vi "Panther Logs for DQMH.vi"() -> ()   [LabVIEW 2016]
uses:
  <resource>/dialog/lvconfig.llb/LV Config Read Boolean.vi
  <resource>/dialog/lvconfig.llb/LV Config Write Boolean.vi
panel:
  in  "Panther Logs":bool
  # "Panther Logs for DQMH®\n\nThis tool creates a file called <PantherLAB_Log.csv> next to the Active LabVIEW Project.\n\nIt will create a log for each executed DQMH task .\n\n\nTo enable/disable logging click the Checkbox."
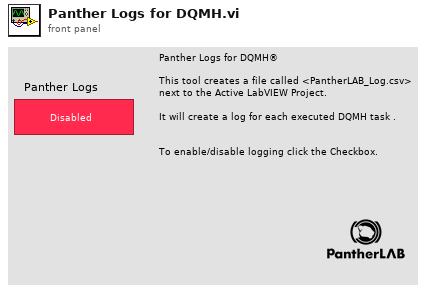
[diagram p1: front panel]
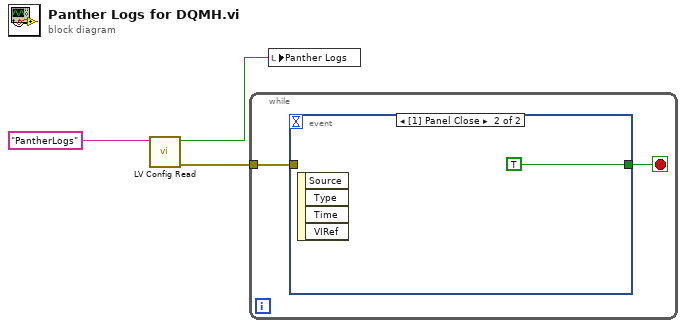
[diagram p0: block diagram]
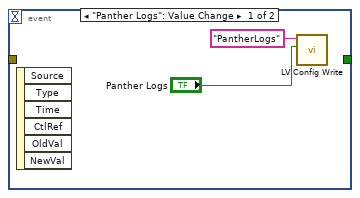
[diagram p2: hidden frame]
diagram:
  n1 = call-poly <resource>:"LV Config Read.vi"("key"="PantherLogs") -> ("error out"=w3:errorcluster, "value"=w1:bool)  [unwired: 4 in, 1 out]
  n2 = while {
    tunnel: w3 -> [w5]
    stop <- w4 stop-if-true
    n3 = event shown="[1] Panel Close" {
      selector: _ -> [_ _]
      dyn-events: _ -> [_ _]
      timeout: _ -> [_ _]
      tunnel: w5 -> [_ _]
      tunnel: [_ TRUE] -> w4
      event "Panther Logs": Value Change {
        n4 = event-data() -> ()  [unwired: 1 in, 6 out]
        n5 = call-poly <resource>:"LV Config Write.vi"("value"="Panther Logs", "key"="PantherLogs") -> ()  [unwired: 5 in, 1 out]
      }
      event Panel Close {
        n6 = event-data() -> ()  [unwired: 1 in, 4 out]
      }
    }
  }
  n7 = local write "Panther Logs"(w1) -> ()
